vi "Source Off Function.vi"(7 "Off Function (DCVOLTS)":T1(ring)=enum."DCAMPS (0 A source)", 8 "error in (no error)":errorcluster, 9 "Channel (Channel A)":T2, 10 "Node In":string, 11 "VISA resource name":refnum<visa-resource-name>) -> (0 "error out":errorcluster, 2 "Node Out":string, 3 "VISA resource name out":refnum<visa-resource-name>, 4 "Command String":string)   [LabVIEW 2013, in "Keithley 2600 Series.lvlib"]
doc: "Source function for the source when the output is off and the SMU is in normal output-off mode. This attribute is only use when the smuX.source.offmode attribute is set to smuX.OUTPUT_NORMAL\n\n<b>Functions and Attributes Used</b>\nsmuX.source.offfunc"
uses:
  Keithley 2600 Series.lvlib
  Private/GlobalVariables.vi
  Channel.ctl
panel:
  # "(c) 2011 Keithley Instruments, Inc.  ALL RIGHTS RESERVED."
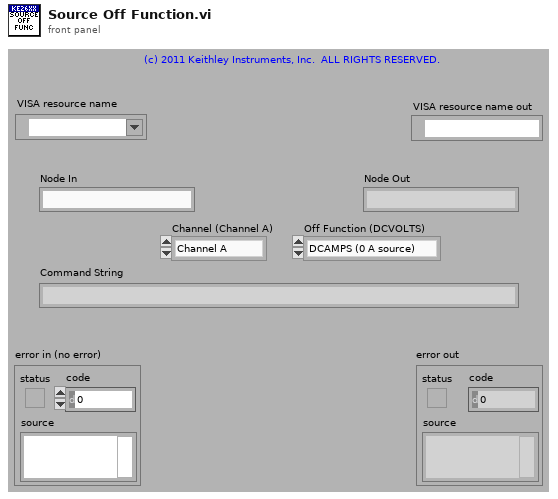
[diagram p1: front panel]
types:
  T1 = enum32{"DCVOLTS (0 V source)", "DCAMPS (0 A source)"}
  T2 = typedef "Keithley 2600 Series.lvlib/Channel.ctl" = enum32{"Channel A", "Channel B"}
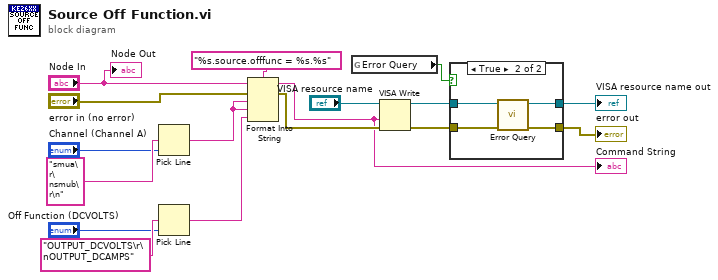
[diagram p0: block diagram]
diagram:
  n1 = Pick Line(multi-line string="smua\r\nsmub\r\n" ("options"), line index="Channel (Channel A)") -> (output string=w4:string)  [unwired: 1 out]
  n2 = Pick Line(multi-line string="OUTPUT_DCVOLTS\r\nOUTPUT_DCAMPS" ("options"), line index="Off Function (DCVOLTS)") -> (output string=w5:string)  [unwired: 1 out]
  n3 = Format Into String(format string="%s.source.offfunc = %s.%s", initial string="Node In", error in="error in (no error)", w4, w4, w5) -> (resulting string=w1:string, error out=w2:errorcluster)
  "Command String" <- w1
  n4 = global read "GlobalVariables.vi" "Error Query"() -> (w13:bool)
  n5 = VISA Write(VISA resource name="VISA resource name", write buffer=w1, error in (no error)=w2) -> (VISA resource name out=w12:refnum<visa-resource-name>, error out=w11:errorcluster)  [unwired: 1 out]
  n6 = case shown="True" w13 {
    tunnel: w12 -> [w19 w23]
    tunnel: w11 -> [w18 w22]
    tunnel: [w19 w21] -> w10
    tunnel: [w18 w20] -> w9
    frame False {
    }
    frame True {
      n7 = call "Error Query.vi"("error in (no error)"=w22, "VISA resource name"=w23) -> ("error out"=w20:errorcluster, "VISA resource name out"=w21:refnum<visa-resource-name>)  [unwired: 8 out]
    }
  }
  "VISA resource name out" <- w10
  "error out" <- w9
  "Node Out" <- "Node In"
